vi "Stop Module.vi"(8 "error in":errorcluster, 9 "Wait for Module to stop? (F)":bool, 10 "Origin":string, 11 "Module ID":i32=-1) -> (0 "error out":errorcluster)   [LabVIEW 2021, in "Slave.lvlib"]
doc: "Send the Stop request to the Module's Main.vi. If <b>Wait for Module to stop?</b> is TRUE, then this VI will not complete execution until the Module Main VI has stopped running.\n\n<b>Note:</b> If the cloneable module is running as singleton, then the 'Wait for Module to stop?' input is ignored... this VI will <b>always</b> wait until a cloneable Main VI running as singleton has stopped running.\n_____\nBased on DQMH Project Template 6.1.0.94.\n\n<b>Note:</b> This VI was modified by the <b>Validate DQMH Module</b> tool to remove the Status Updated.vi subVI call."
uses:
  Slave.lvlib
  Stop Argument--cluster.ctl
  Module Running State--enum.ctl
  Main.vi
  <vilib>/DQMH Consortium/Lumos API/Libraries/SDV API/SDV API.lvlib
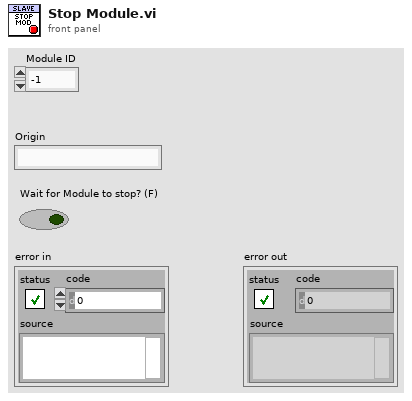
[diagram p1: front panel]
types:
  T1 = typedef "Slave.lvlib/Module Running State--enum.ctl" = enum16{"Not Running", "Running as Cloneable", "Running as Singleton"}
  T2 = typedef "Slave.lvlib/Stop Argument--cluster.ctl" = cluster{"Module ID":i32, "Origin":string, "Exit via Stop Module Req?":bool, "Wait for Module to stop?":bool}
  T3 = typedef "Slave.lvlib/Request Events--cluster.ctl" = cluster{"Stop Module":refnum<user-event>, "Show Panel":refnum<user-event>, "Hide Panel":refnum<user-event>, "Show Diagram":refnum<user-event>, "Get Module Execution Status":refnum<user-event>}
  T4 = enum32{"Bad", "Idle", "Run top level", "Running"}
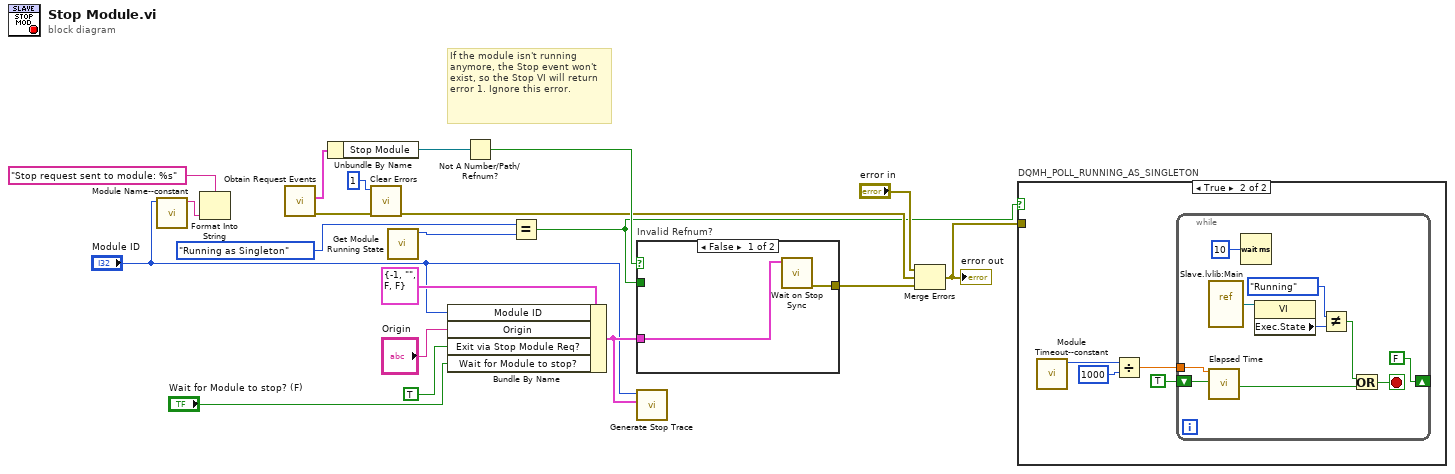
[diagram p0: block diagram]
diagram:
  # "If the module isn't running anymore, the Stop event won't exist, so the Stop VI will return error 1. Ignore this error."
  n1 = call "Module Name--constant.vi"("Module ID"="Module ID") -> ("Module Name"=w18:string)  [unwired: 10 in]
  n2 = Format Into String(format string="Stop request sent to module: %s", w18) -> ()  [unwired: 2 in, 2 out]
  n3 = call "Obtain Request Events.vi"() -> ("error out"=w12:errorcluster, "Slave Request Events"=w10:T3)  [unwired: 10 in]
  n4 = Unbundle By Name(w10) -> ("Stop Module"=w14:refnum<user-event>)
  n5 = call <vilib>:"Clear Errors.vi"("error in (no error)"=w12, "specific error code to clear (0: all)"=1) -> ("error out"=w9:errorcluster)  [unwired: 4 in, 1 out]
  n6 = call "Get Module Running State.vi"() -> ("Module Running State"=w5:T1)  [unwired: 11 in]
  n7 = Bundle By Name(cluster=T2 {"Module ID"=-1, "Origin"="", "Exit via Stop Module Req?"=FALSE, "Wait for Module to stop?"=FALSE} ("event data"), "Module ID"="Module ID", "Origin"="Origin", "Exit via Stop Module Req?"=TRUE, "Wait for Module to stop?"="Wait for Module to stop? (F)") -> (w13:T2)
  n8 = Not A Number/Path/Refnum?(number/path/refnum=w14) -> (NaN/Path/Refnum?=w15:bool)
  n9 = Equal?(x=Module_Running_State--enum."Running as Singleton", y=w5) -> (x = y?=w4:bool)
  n10 = case "Invalid Refnum?" shown="False" w15 {
    tunnel: [w22 _] -> w8
    tunnel: w13 -> [w21 _]
    tunnel: w4 -> [_ _]
    frame False {
      n11 = call "Wait on Stop Sync.vi"("Stop Argument"=w21) -> ("error out"=w22:errorcluster)  [unwired: 10 in]
    }
    frame True {
      # "Module is exiting. No need to send the standard \"not running\" error that is sent in other request VIs."
    }
  }
  n12 = call <vilib>:"Generate Stop Trace.vi"("Payload"=w13, "Module ID (0)"="Module ID") -> ()  [unwired: 9 in, 1 out]
  n13 = Merge Errors("error in", w9, w8) -> (w2:errorcluster)
  "error out" <- w2
  n14 = case "DQMH_POLL_RUNNING_AS_SINGLETON" shown="True" w4 {
    tunnel: w2 -> [_ _]
    frame False {
    }
    frame True {
      n15 = call "Module Timeout--constant.vi"() -> ("Module Timeout"=w26:i32)  [unwired: 11 in]
      n16 = Divide(x=w26, y=1000) -> (x/y=w24:dbl)
      n17 = while {
        tunnel: w24 -> [w29]
        shift-right: [FALSE] -> _
        shift-left: TRUE -> [w30]
        stop <- w32 stop-if-true
        n18 = vi-ref "Slave.lvlib:Main.vi"() -> (w36:refnum<vi>)
        n19 = call "Elapsed Time"("Time Target (s)"=w29, "Reset"=w30) -> ("Time has Elapsed"=w28:bool)  [unwired: 10 in, 7 out]
        n20 = Wait (ms)(milliseconds to wait=u32 10) -> ()  [unwired: 1 out]
        n21 = property on="Property Node" class="VI"(reference=w36) -> ("Exec.State"=w35:T4)  [unwired: 1 in, 2 out]
        n22 = Not Equal?(x=T4."Running", y=w35) -> (x != y?=w33:bool)
        n23 = Or(x=w33, y=w28) -> (x .or. y?=w32:bool)
      }
    }
  }
